vi "hardware_apply_settings.vi"(8 "error in (no error)":errorcluster, 11 "hydraharp in":refnum<class "picoharp.lvclass">) -> (0 "error out":errorcluster, 3 "hydraharp out":refnum<class "picoharp.lvclass">)   [LabVIEW 2015, in "picoharp.lvclass"]
uses:
  picoharp.lvclass
  picoharp.lvclass/picoharp.ctl
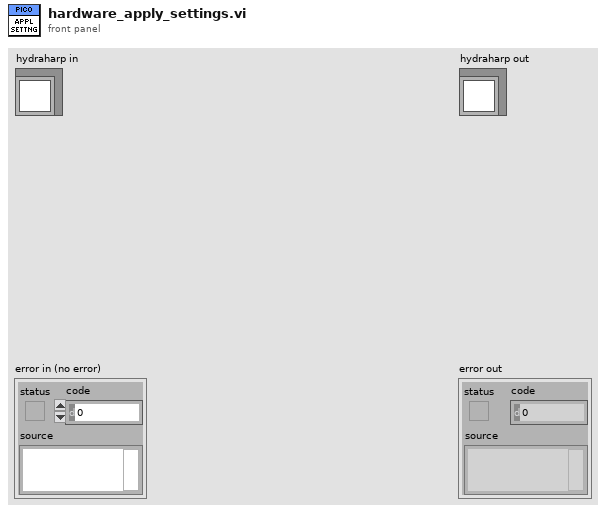
[diagram p1: front panel]
types:
  T1 = typedef "hpanel_sync_settings.ctl" = cluster{"snc_count":i32, "snc_level":i32, "snc_ZeroX":i32, "snc_offs":i32, "sync_div":T2}
  T2 = typedef "hpanel_sync_div.ctl" = enum16{"1", "2", "4", "8"}
  T3 = typedef "hpanel_channel_settings.ctl" = cluster{"ch_counts":i32, "ch_level":i32, "ch_ZeroX":i32, "ch_offs":i32}
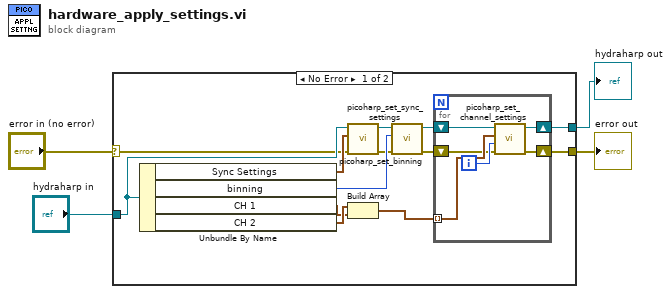
[diagram p0: block diagram]
diagram:
  n1 = case shown="No Error" "error in (no error)" {
    selector: "error in (no error)" -> [w9 w24]
    tunnel: "hydraharp in" -> [w17 w25]
    tunnel: [w8 w25] -> w2
    tunnel: [w7 w24] -> w1
    frame No Error {
      n2 = Unbundle By Name(w17) -> ("Sync Settings"=w16:T1, "binning"=w14:i32, "CH 1"=w5:T3, "CH 2"=w6:T3)
      n3 = call "picoharp_set_sync_settings.vi"("error in (no error)"=w9, "sync_settings"=w16, "hydraharp in"=w17) -> ("error out"=w10:errorcluster, "hydraharp out"=w15:refnum<class "picoharp.lvclass">)  [unwired: 7 in]
      n4 = Build Array(w6, w5) -> (w12:T3[])
      n5 = call "picoharp_set_binning.vi"("error in (no error)"=w10, "Binning"=w14, "hydraharp in"=w15) -> ("error out"=w11:errorcluster, "hydraharp out"=w13:refnum<class "picoharp.lvclass">)  [unwired: 7 in]
      n6 = for {
        shift-right: [w22] -> w8
        shift-left: w13 -> [w23]
        tunnel: w12 -> [w21] mode=indexing
        shift-right: [w18] -> w7
        shift-left: w11 -> [w19]
        i -> [w20]
        n7 = call "picoharp_set_channel_settings.vi"("error in (no error)"=w19, "channel"=w20, "ch_settings"=w21, "hydraharp in"=w23) -> ("error out"=w18:errorcluster, "hydraharp out"=w22:refnum<class "picoharp.lvclass">)  [unwired: 6 in]
      }
    }
    frame Error {
    }
  }
  "error out" <- w1
  "hydraharp out" <- w2
